vi "Read Configuration Data.vi"(0 "Path":path, 3 "error in (no error)":errorcluster) -> (8 "Configuration Settings":T1={"Signal type"=enum."Sine Wave", "Amplitude"=1.0, "Offset"=0.0, "Amplitude 2"=1.0, "Frequency"=10.0} {"Frequency" format="%0.2p"; "Amplitude 2" format="%.2p"; "Offset" format="%0.2p"; "Amplitude" format="%0.2p"}, 10 "error out":errorcluster)   [LabVIEW 2022 SP3]
uses:
  controls/Configuration Settings.ctl
  <vilib>/Utility/config.llb/Read Key (U32).vi
  <vilib>/Utility/config.llb/Read Key (Double).vi
  <vilib>/Utility/config.llb/NI_LVConfig.lvlib
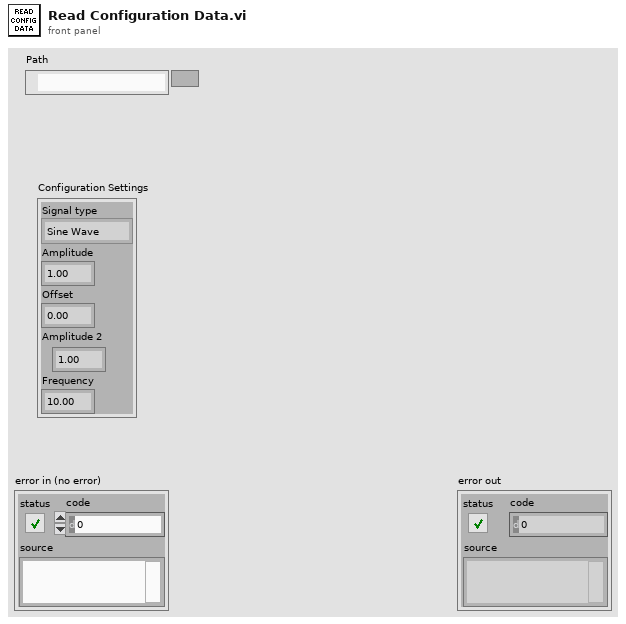
[diagram p1: front panel]
types:
  T1 = typedef "Configuration Settings.ctl" = cluster{"Signal type":enum16{"Sine Wave", "Triangle Wave", "Square Wave", "Sawtooth Wave"}, "Amplitude":dbl, "Offset":dbl, "Amplitude 2":dbl, "Frequency":dbl}
  T2 = enum16{"Sine Wave", "Triangle Wave", "Square Wave", "Sawtooth Wave"}
  T3 = typedef "NI_LVConfig.lvlib/Config Data RefNum.ctl" = refnum<k1>
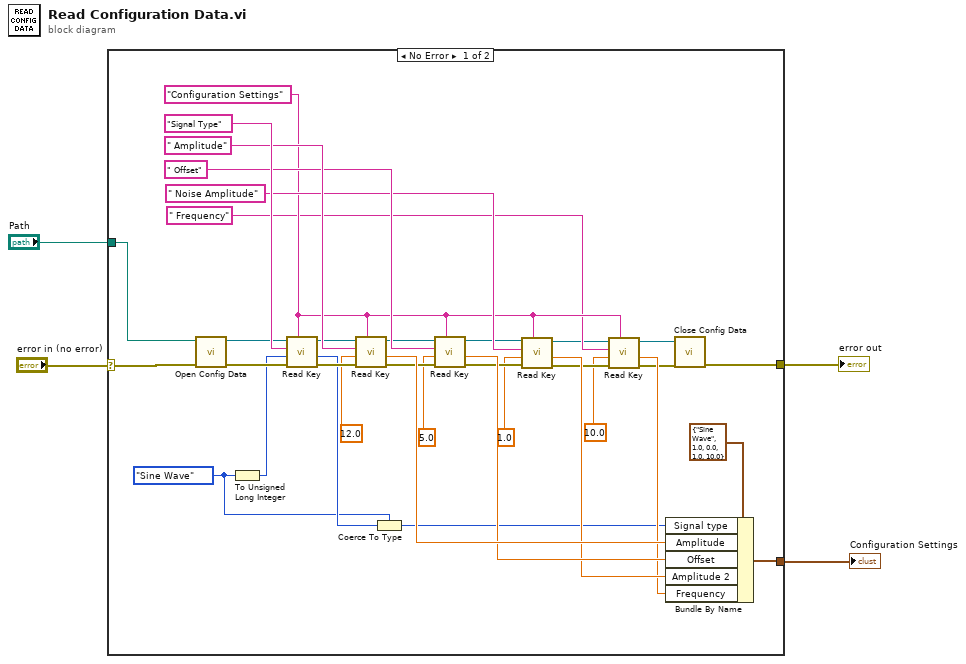
[diagram p0: block diagram]
diagram:
  n1 = case shown="No Error" "error in (no error)" {
    selector: "error in (no error)" -> [w39 _]
    tunnel: [w35 _] -> w3
    tunnel: "Path" -> [w38 _]
    tunnel: [w36 _] -> w1
    frame No Error {
      w9 = T2."Sine Wave" ("Signal type")
      w23 = "Configuration Settings"
      n2 = call <vilib>:"Open Config Data.vi"("error in (no error)"=w39, "configuration file path"=w38) -> ("error out"=w18:errorcluster, "refnum"=w31:T3)  [unwired: 7 in, 1 out]
      n3 = To Unsigned Long Integer(number=w9) -> (unsigned 32bit integer=w10:u32)
      n4 = call-poly <vilib>:"Read Key.vi"("section"=w23, "error in (no error)"=w18, "default value"=w10, "key"="Signal Type", "refnum"=w31) -> ("error out"=w17:errorcluster, "value"=w11:u32, "refnum out"=w28:T3)  [unwired: 3 in, 1 out]
      n5 = call-poly <vilib>:"Read Key.vi"("section"=w23, "error in (no error)"=w17, "default value"=12.0, "key"=" Amplitude", "refnum"=w28) -> ("error out"=w16:errorcluster, "value"=w32:dbl, "refnum out"=w27:T3)  [unwired: 3 in, 1 out]
      n6 = Coerce To Type(0:w11, 1:w9) -> (2:w12:T2)
      n7 = call-poly <vilib>:"Read Key.vi"("section"=w23, "error in (no error)"=w16, "default value"=5.0, "key"=" Offset", "refnum"=w27) -> ("error out"=w15:errorcluster, "value"=w29:dbl, "refnum out"=w24:T3)  [unwired: 3 in, 1 out]
      n8 = call-poly <vilib>:"Read Key.vi"("section"=w23, "error in (no error)"=w15, "default value"=1.0, "key"=" Noise Amplitude", "refnum"=w24) -> ("error out"=w14:errorcluster, "value"=w25:dbl, "refnum out"=w20:T3)  [unwired: 3 in, 1 out]
      n9 = call-poly <vilib>:"Read Key.vi"("section"=w23, "error in (no error)"=w14, "default value"=10.0, "key"=" Frequency", "refnum"=w20) -> ("error out"=w13:errorcluster, "value"=w21:dbl, "refnum out"=w19:T3)  [unwired: 3 in, 1 out]
      n10 = Bundle By Name(cluster=T1 {"Signal type"=enum."Sine Wave", "Amplitude"=1.0, "Offset"=0.0, "Amplitude 2"=1.0, "Frequency"=10.0} ("Configuration Settings"), "Signal type"=w12, "Amplitude"=w32, "Offset"=w29, "Amplitude 2"=w25, "Frequency"=w21) -> (w36:T1)
      n11 = call <vilib>:"Close Config Data.vi"("error in (no error)"=w13, "refnum"=w19) -> ("error out"=w35:errorcluster)  [unwired: 8 in, 1 out]
    }
    frame Error {
    }
  }
  "error out" <- w3
  "Configuration Settings" <- w1
